vi "Read.vi"(0 "System Interface in":refnum<class "System Interface.lvclass">, 11 "Error In":errorcluster) -> (4 "System Interface out":refnum<class "System Interface.lvclass">, 6 "Process Data":T1, 15 "Error Out":errorcluster)   [LabVIEW 2020, in "Waveform(DBL) Array.lvlib"]
uses:
  <vilib>/ADAS Record/CustomDataTypes/Waveform(DBL) Array/Waveform(DBL) Array.lvlib
  <vilib>/FlexLogger/SDK/PluginSDK.lvlibp/PEFClasses/SDK/System Interface/System Interface.lvclass
  <vilib>/ADAS Record/CustomDataTypes/Waveform(DBL) Array/Process Data.ctl
  4520f411-daba-4182-bc35-841ea590f987.vi
  4520f411-daba-4182-bc35-841ea590f987.vi/200e1971-199f-4368-bba3-f4cf81656045.vi
  4520f411-daba-4182-bc35-841ea590f987.vi/0dd6222d-dbf1-4022-9e9c-a30c51012c18.vi
  <vilib>/Utility/error.llb/Clear Errors.vi
  4520f411-daba-4182-bc35-841ea590f987.vi/200e1971-199f-4368-bba3-f4cf81656045.vi/2099ef80-a8f9-4b1c-a5c6-b23612a5eac4.vi
  4520f411-daba-4182-bc35-841ea590f987.vi/0dd6222d-dbf1-4022-9e9c-a30c51012c18.vi/7bf3da57-5b1d-4b21-896d-7766261ce726.vi
  4520f411-daba-4182-bc35-841ea590f987.vi/0dd6222d-dbf1-4022-9e9c-a30c51012c18.vi/3b588064-68fc-43f0-9f28-230c287437e0.vi
  <vilib>/FlexLogger/TestSystemInterface/Test System Interface.lvclass
  C:/Program Files/National Instruments/LabVIEW 2020/vi.lib/FlexLogger/SDK/PluginSDK.lvlibp/PEFClasses/SDK/System Interface/System Interface.lvclass
  <vilib>/ADAS Record/CustomData/_Custom_RegisterType.vi
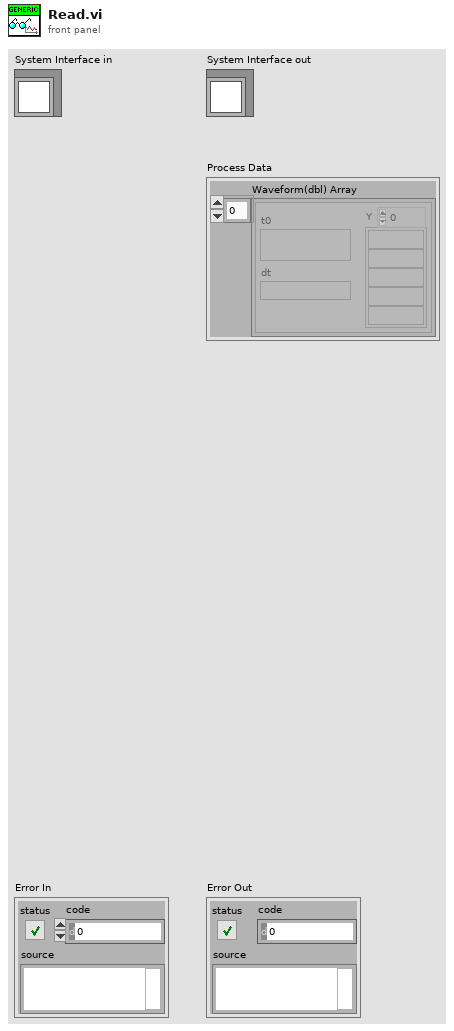
[diagram p1: front panel]
types:
  T1 = typedef "Waveform(DBL) Array.lvlib/Process Data.ctl" = cluster{"Waveform(dbl) Array":waveform(dbl)[]}
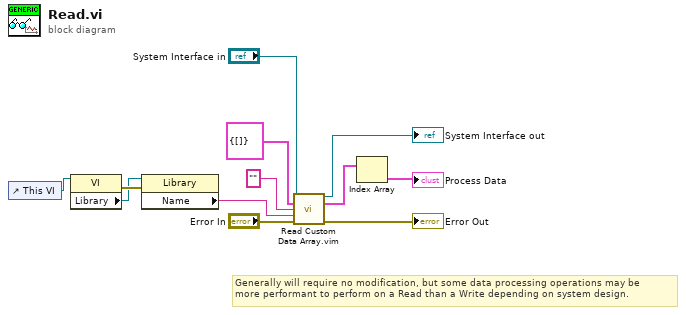
[diagram p0: block diagram]
diagram:
  # "Generally will require no modification, but some data processing operations may be\nmore performant to perform on a Read than a Write depending on system design."
  n1 = control-ref of="This VI"() -> (w4:refnum<vi>)
  n2 = property class="VI"(reference=w4) -> (error out=w3:errorcluster, "Library"=w2:refnum<vi>)  [unwired: 1 in, 1 out]
  n3 = property class="Library"(reference=w2, error in=w3) -> ("Name"=w1:string)  [unwired: 2 out]
  n4 = call "Read Custom Data Array.vim"("System Interface"="System Interface in", "Data Element Type"=T1 {"Waveform(dbl) Array"=[]} ("Process Data"), "Metadata Element Type"="" ("appended array"), "Type"=w1, "error in (no error)"="Error In") -> ("System Interface out"=→"System Interface out":refnum<class "System Interface.lvclass">, "Data Array"=w5:T1[], "error out"=→"Error Out":errorcluster)  [unwired: 4 in, 4 out]
  n5 = Index Array(array=w5) -> (element=→"Process Data":T1)  [unwired: 1 in]
